vi "Change State.vi"(8 "error in":errorcluster, 10 "instr state":T1, 11 "Instrument in":refnum<class "Instrument.lvclass">) -> (0 "error out":errorcluster, 3 "Instrument out":refnum<class "Instrument.lvclass">)   [LabVIEW 2018, in "Instrument.lvclass"]
doc: "This VI is used to enqueue a new state for the Instrument state machine."
uses:
  Instrument.lvclass
  state.ctl
  Instrument.lvclass/Instrument.ctl
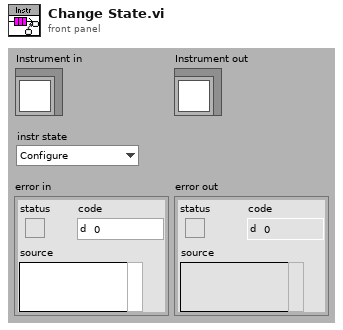
[diagram p1: front panel]
types:
  T1 = typedef "Instrument.lvclass/state.ctl" = enum8{"Configure", "Acquire", "Wait", "Quit", "Handle Error", "NOOP"}
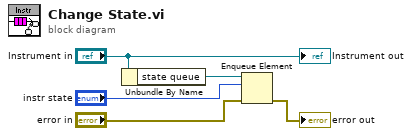
[diagram p0: block diagram]
diagram:
  n1 = Unbundle By Name("Instrument in") -> ("state queue"=w1:refnum<queue>)
  n2 = Enqueue Element(queue=w1, element="instr state", error in (no error)="error in") -> (error out=→"error out":errorcluster)  [unwired: 1 in, 2 out]
  "Instrument out" <- "Instrument in"
